vi "FRCts20_Backend_Dyn_GetOpenTeams.vi"(6 "Message Attributes":T4, 8 "error in (no error)":errorcluster, 10 "Data":string, 11 "Engine_Refnums":T1) -> (0 "error out":errorcluster)   [LabVIEW 2014, in "FRCts20_Backend_DynamicLoad.lvlib"]
doc: "Gets list of teams that do not have SW associated with them"
uses:
  FRCts20_Backend_DynamicLoad.lvlib
  Dependencies/Keyed Array/KeyedArray.ctl
  Dependencies/Keyed Array/Tools_KeyedArray.lvlib
  Dependencies/AMC/_SubVIs/TypeDefs/Message.ctl
  Dependencies/AMC/AMC.lvlib
  Dependencies/AMC/_SubVIs/TypeDefs/Message Queue.ctl
  FRCts20_Backend_EngineRefnums.ctl
  FRCts20_Backend_Engine.lvlib
  <vilib>/addons/database/Connection.llb/Conn ObjectReference.ctl
  <vilib>/addons/database/NI_Database_API.lvlib
  INI_Accessor/FRCts20_Backend_INI Controller.lvclass
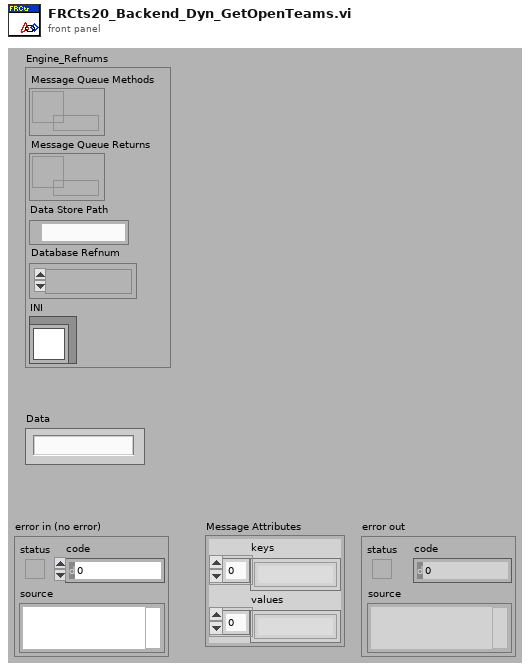
[diagram p1: front panel]
types:
  T1 = typedef "FRCts20_Backend_Engine.lvlib/FRCts20_Backend_EngineRefnums.ctl" = cluster{"Message Queue Methods":T2, "Message Queue Returns":T2, "Data Store Path":path, "Database Refnum":T3, "INI":refnum<class "FRCts20_Backend_INI Controller.lvclass">}
  T2 = typedef "AMC.lvlib/Message Queue.ctl" = refnum<queue>
  T3 = typedef "NI_Database_API.lvlib/Conn ObjectReference.ctl" = refnum<k1>
  T4 = typedef "Tools_KeyedArray.lvlib/KeyedArray.ctl" = cluster{"keys":string[], "values":string[]}
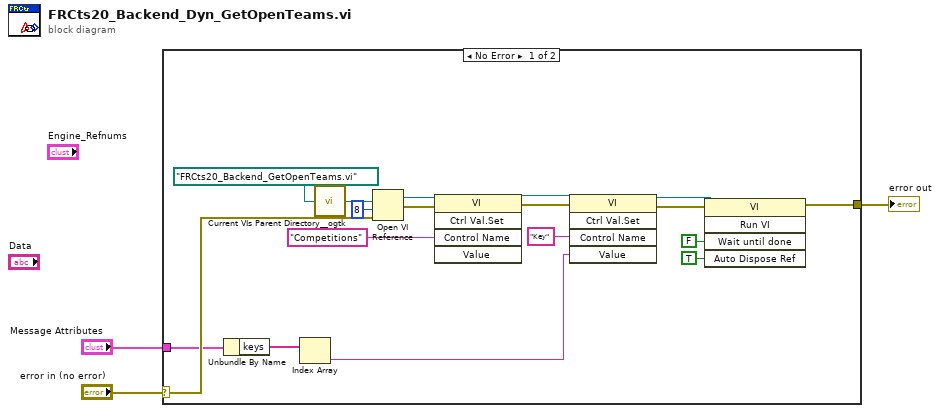
[diagram p0: block diagram]
diagram:
  n1 = case shown="No Error" "error in (no error)" {
    selector: "error in (no error)" -> [w19 w22]
    tunnel: [w8 w22] -> w2
    tunnel: "Message Attributes" -> [w6 _]
    frame No Error {
      n2 = Unbundle By Name(w6) -> ("keys"=w5:string[])
      n3 = Index Array(array=w5) -> (element=w4:string)  [unwired: 1 in]
      n4 = call "Current VIs Parent Directory__ogtk.vi"("Relative path (.)"=path "FRCts20_Backend_GetOpenTeams.vi") -> ("Parent Directory (+ Relative)"=w20:path)  [unwired: 4 in]
      n5 = Open VI Reference(vi path=w20, options=8, error in (no error)=w19) -> (vi reference=w18:refnum<vi>, error out=w17:errorcluster)  [unwired: 3 in]
      n6 = invoke class="VI" method="Ctrl Val.Set"(reference=w18, error in=w17, "Control Name"="Competitions") -> (reference out=w15:refnum<vi>, error out=w14:errorcluster)  [unwired: 2 in, 3 out]
      n7 = invoke class="VI" method="Ctrl Val.Set"(reference=w15, error in=w14, "Control Name"="Key", "Value"=w4) -> (reference out=w9:refnum<vi>, error out=w10:errorcluster)  [unwired: 1 in, 3 out]
      n8 = invoke class="VI" method="Run VI"(reference=w9, error in=w10, "Wait until done"=FALSE ("Wait Until Done"), "Auto Dispose Ref"=TRUE ("Auto Dispose Reference")) -> (error out=w8:errorcluster)  [unwired: 1 in, 4 out]
    }
    frame Error {
    }
  }
  "error out" <- w2
